vi "StartUpSequence.vi"(0 "Tab Control":enum32{"General"}(tab), 2 "error in (no error)":errorcluster, 3 "Cams":enum32{"Point", "Area", "ROI"}(tab), 4 "IntGraph Refnum":refnum<vi>, 5 "TabCtl Refnum 2":refnum<vi>, 6 "Str Refnum":refnum<vi>, 7 "TabCtl Refnum":refnum<vi>) -> (1 "error out 2":errorcluster)   [LabVIEW 2011]
panel:
  out "Point":dbl[][](graph)
  out "Area":i32[][](graph)
  in  "Confocal Mode Area Image calculation":enum32{"Maximum", "Average", "Normalized"}(radio)
  in  "colorArea":enum32{"Red", "Green", "Blue"}(radio)
  in  "Emergency Exit":bool
  out "Terminal":string
  in  "Start Measurement":bool
  in  "Clear Terminal":bool
  out "Interlock":bool
  out "Laser":bool
  out "Scanning":bool
  out "Config":bool
  out "Device":bool
  in  "Camera Settings":bool
  in  "AOTF Settings":bool
  in  "Set Picture":bool
  in  "Move Scanner":bool
  in  "Move Mirror":bool
  in  "Set Workspace":bool
  in  "Laser Power":dbl(slide) min=0.0 max=100.0 step=1.0 scale=0.0..100.0
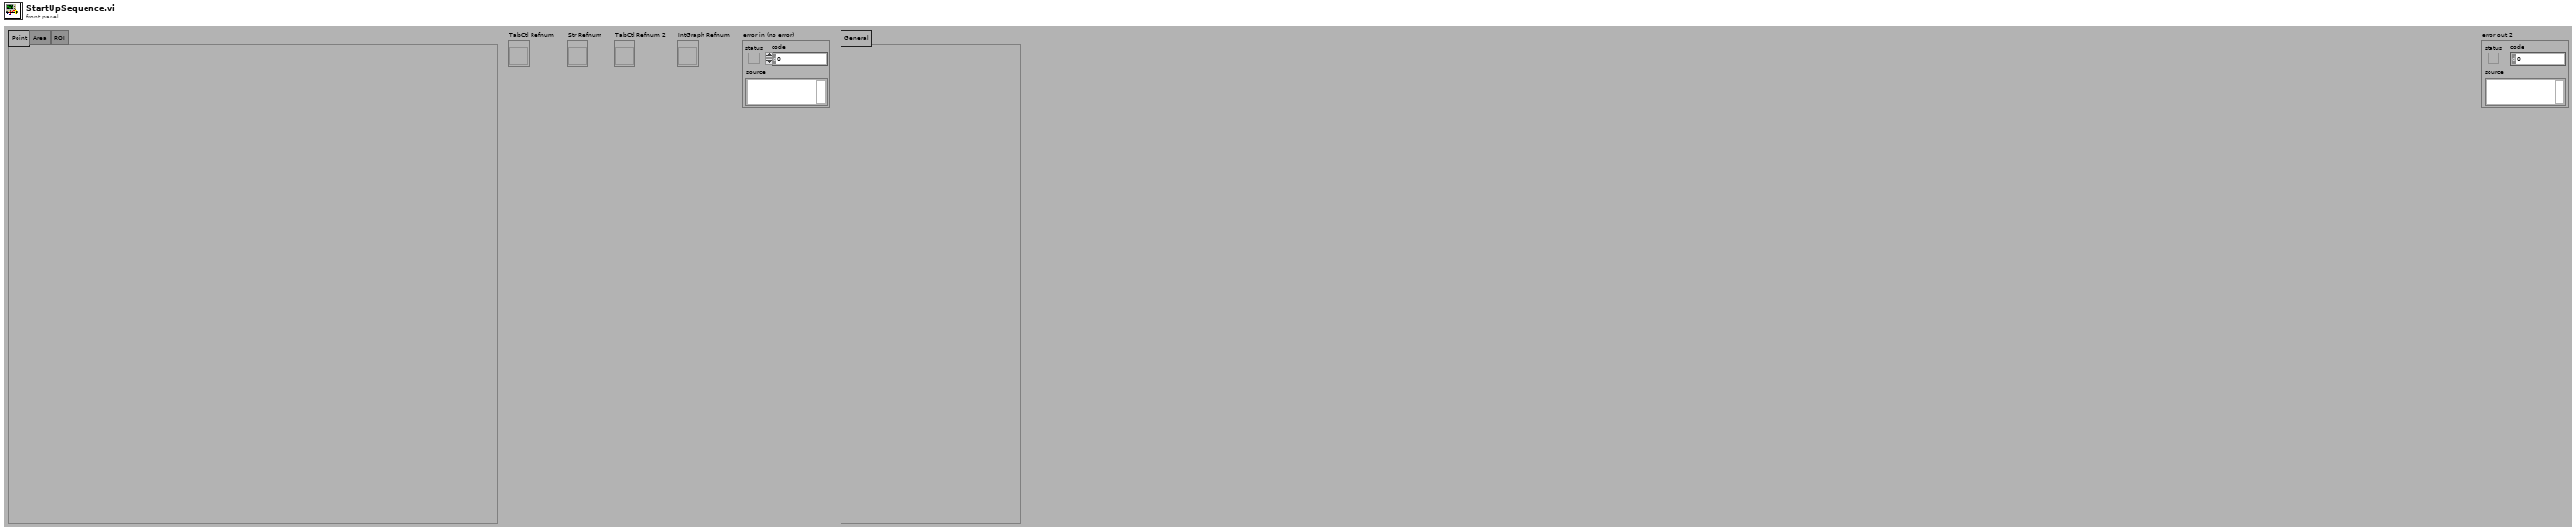
[diagram p1: front panel]
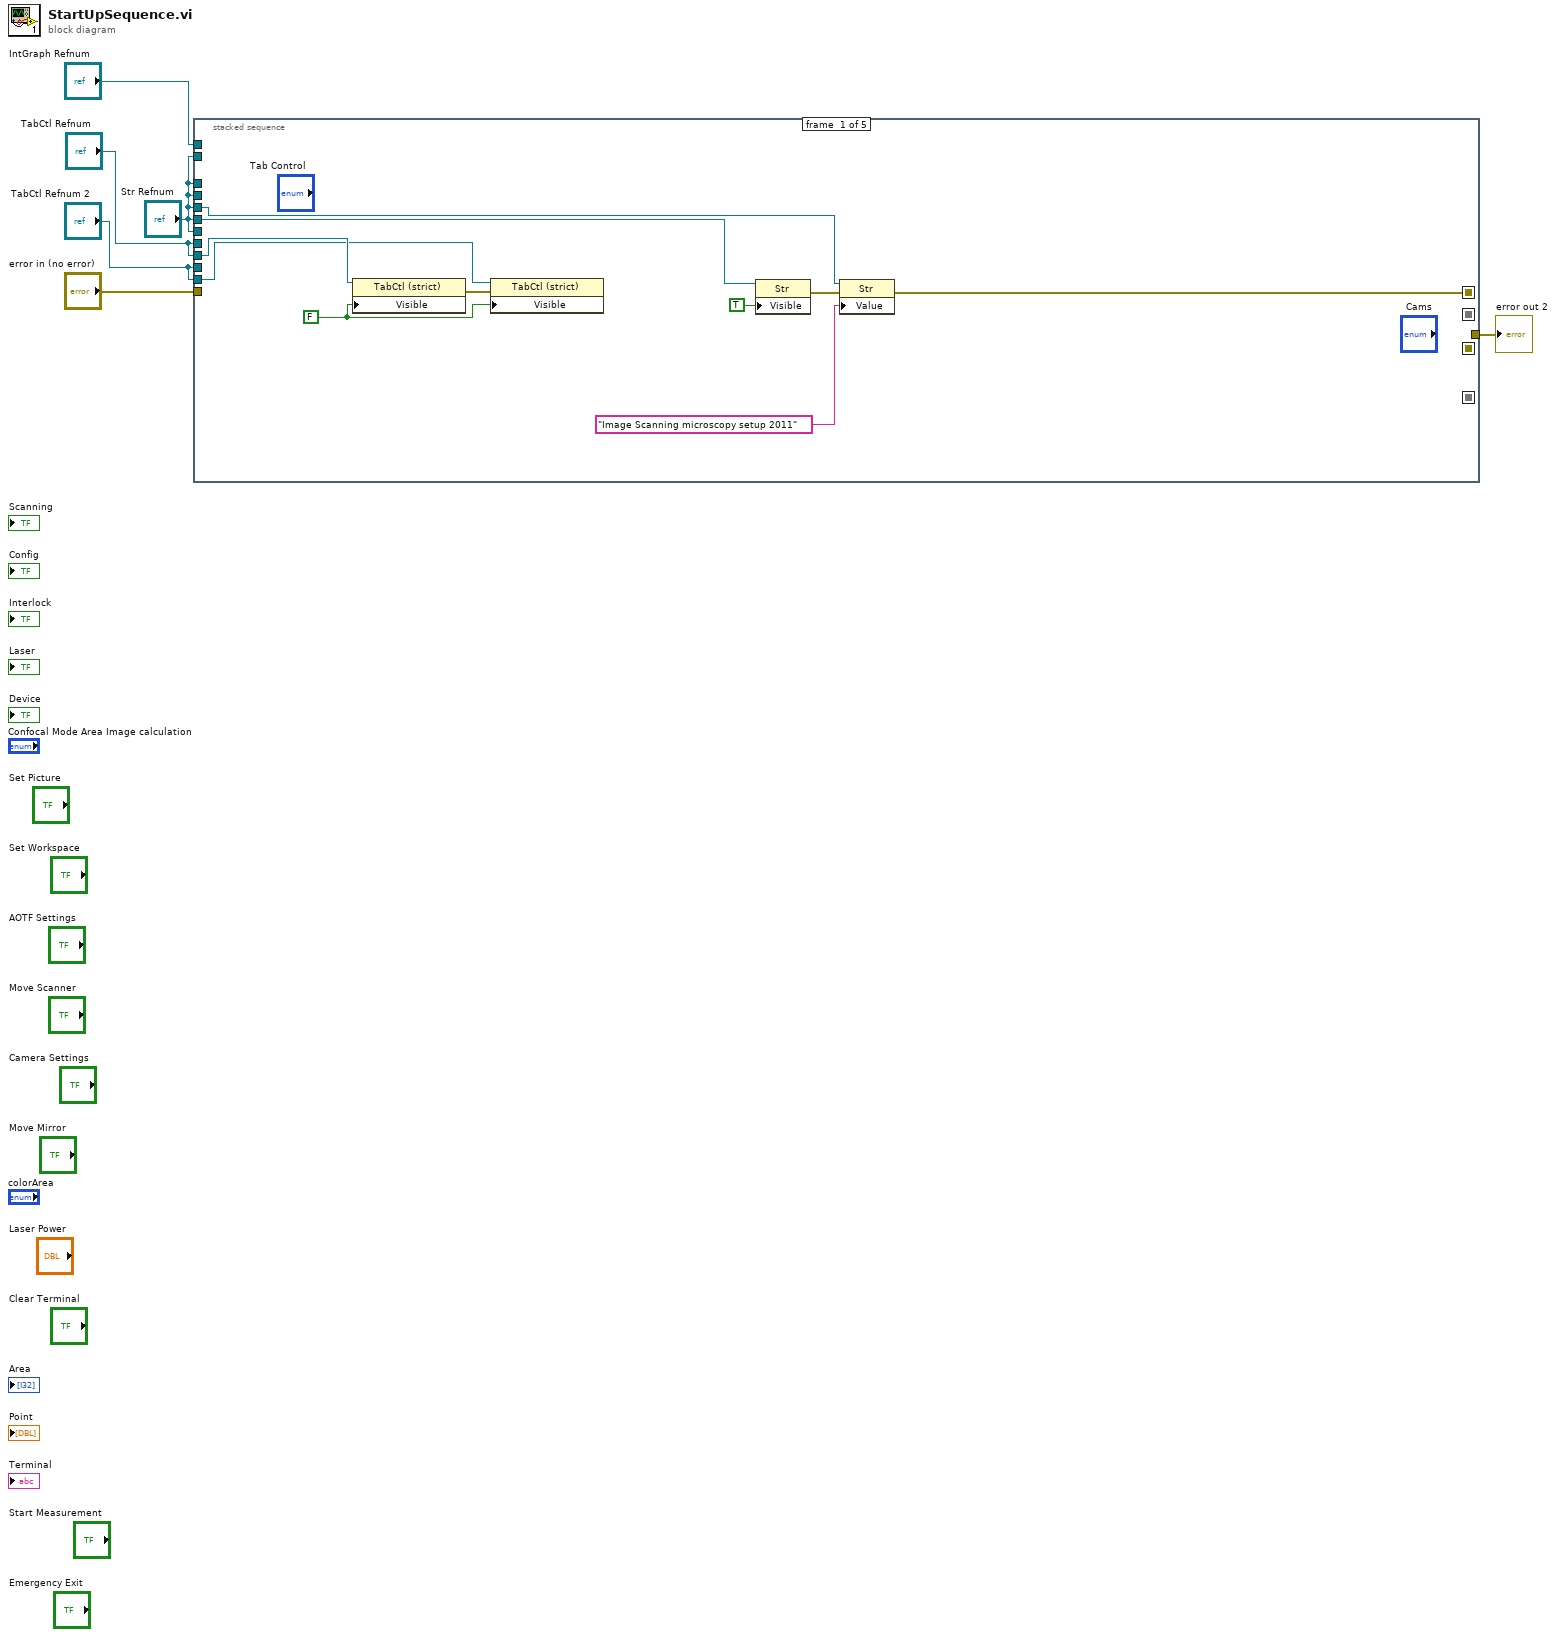
[diagram p0: block diagram]
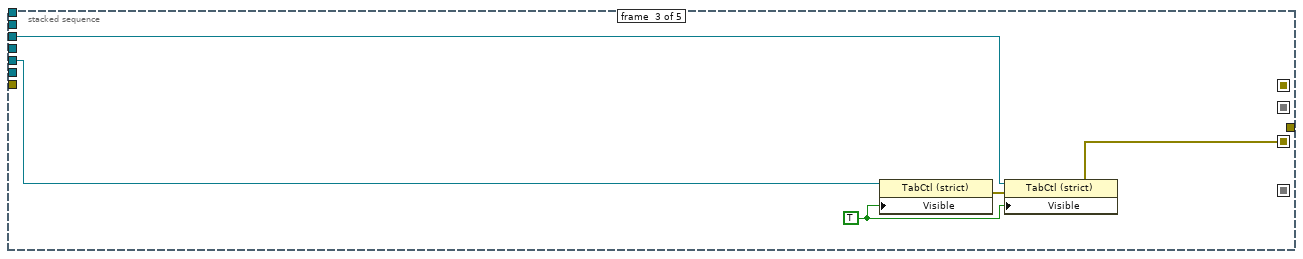
[diagram p3: hidden frame]
diagram:
  n1 = stacked-sequence {
    seq-local: [w18 _ _ _ _] -> [_ _ _ _ _]
    seq-local: [_ _ _ _ _] -> [_ _ w21 _ _]
    tunnel: "error in (no error)" -> [_ _ _ _ _]
    tunnel: [_ _ _ _ _] -> w6
    tunnel: "TabCtl Refnum" -> [w10 _ _ _ _]
    tunnel: "Str Refnum" -> [w9 _ _ _ _]
    tunnel: "TabCtl Refnum 2" -> [w8 _ _ _ _]
    tunnel: "Str Refnum" -> [w7 _ _ _ _]
    tunnel: "Str Refnum" -> [_ _ _ _ _]
    tunnel: "TabCtl Refnum" -> [_ _ w20 _ _]
    tunnel: "TabCtl Refnum 2" -> [_ _ w19 _ _]
    tunnel: "Str Refnum" -> [_ _ _ _ _]
    tunnel: "Str Refnum" -> [_ _ _ _ _]
    tunnel: "Str Refnum" -> [_ _ _ _ _]
    tunnel: "IntGraph Refnum" -> [_ _ _ _ _]
    frame #0 {
      w14 = FALSE ("Visible")
      n2 = property on="Property Node" class="TabCtl (strict)"(reference=w10, "Visible"=w14) -> (error in=w16:errorcluster, error out=w15:errorcluster)  [unwired: 1 out]
      n3 = property on="Property Node" class="TabCtl (strict)"(reference=w8, error in=w15, "Visible"=w14) -> ()  [unwired: 2 out]
      n4 = property on="Property Node" class="Str"(reference=w7, "Visible"=TRUE) -> (error in=w13:errorcluster, error out=w12:errorcluster)  [unwired: 1 out]
      n5 = property on="Property Node" class="Str"(reference=w9, error in=w12, "Value"="Image Scanning microscopy setup 2011" ("Terminal")) -> (error out=w18:errorcluster)  [unwired: 1 out]
    }
    frame #1 {
    }
    frame #2 {
      w22 = TRUE ("Visible")
      n6 = property on="Property Node" class="TabCtl (strict)"(reference=w19, error in=w21, "Visible"=w22) -> (error out=w23:errorcluster)  [unwired: 1 out]
      n7 = property on="Property Node" class="TabCtl (strict)"(reference=w20, error in=w23, "Visible"=w22) -> ()  [unwired: 2 out]
    }
    frame #3 {
    }
    frame #4 {
    }
  }
  "error out 2" <- w6
